vi "Create.vi"(8 "error in (no error)":errorcluster, 11 "obj":refnum<class "Racer.lvclass">) -> (0 "error out":errorcluster, 3 "obj out":refnum<class "Racer.lvclass">)   [LabVIEW 2019, in "Racer.lvclass"]
doc: "Creates an active by ref object.\n\nwww.sciware.com.au\nBSD License (http://www.opensource.org/licenses/bsd-license.php)"
uses:
  Racer.lvclass
  Private/DataMembers.ctl
  Racer.lvclass/Racer.ctl
  Bike/Bike.lvclass
panel:
  in  "data members (type)":T1
  # "BSD License (http://www.opensource.org/licenses/bsd-license.php)"
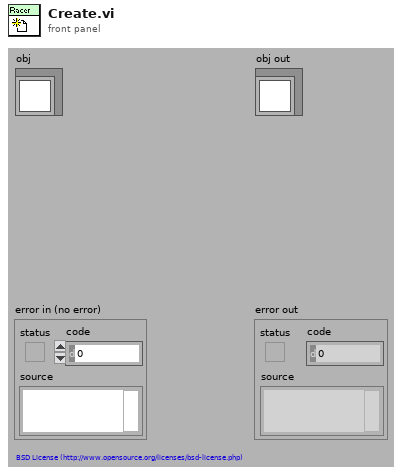
[diagram p1: front panel]
types:
  T1 = typedef "Racer.lvclass/DataMembers.ctl" = cluster{"gear":i32}
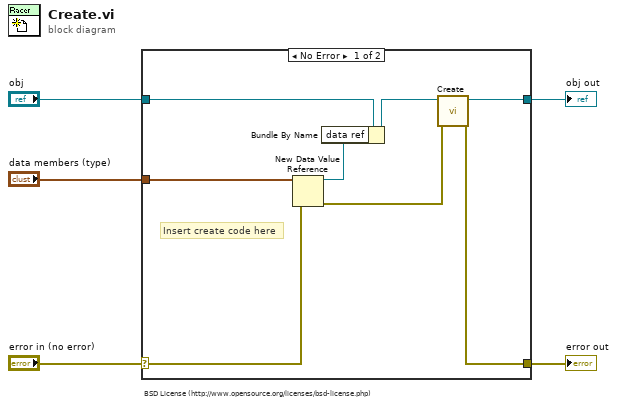
[diagram p0: block diagram]
diagram:
  # "BSD License (http://www.opensource.org/licenses/bsd-license.php)"
  n1 = case shown="No Error" "error in (no error)" {
    selector: "error in (no error)" -> [w13 w15]
    tunnel: [w6 w15] -> w4
    tunnel: "data members (type)" -> [w11 _]
    tunnel: [w7 w14] -> w2
    tunnel: "obj" -> [w10 w14]
    frame No Error {
      # "Insert create code here"
      n2 = New Data Value Reference(data value=w11, error in=w13) -> (data value reference=w12:refnum<data-value>, error out=w8:errorcluster)
      n3 = Bundle By Name(cluster=w10, "data ref"=w12) -> (w9:refnum<class "Racer.lvclass">)
      n4 = call-parent "Create.vi"("error in (no error)"=w8, "obj"=w9) -> ("error out"=w6:errorcluster, "obj out"=w7:refnum<class "Racer.lvclass">)  [unwired: 8 in]
    }
    frame Error {
    }
  }
  "error out" <- w4
  "obj out" <- w2
